vi "Ctr_FindRef[].vi"(5 "加入前缀(空)":string, 7 "ClassName(ALL)":string(combo), 8 "error in":errorcluster, 9 "结束字符串(_%)":string="_%", 10 "CtrlName[]":string[](array[string]), 11 "vi*(Current VI)":refnum<vi>) -> (0 "error out":errorcluster, 1 "CtrlLables[]":string[](array[string]), 2 "ctrls":refnum<vi>[](array[refnum]), 3 "vi* out":refnum<vi>)   [LabVIEW 2016]
uses:
  <vilib>/regexp/Match Regular Expression.xnode
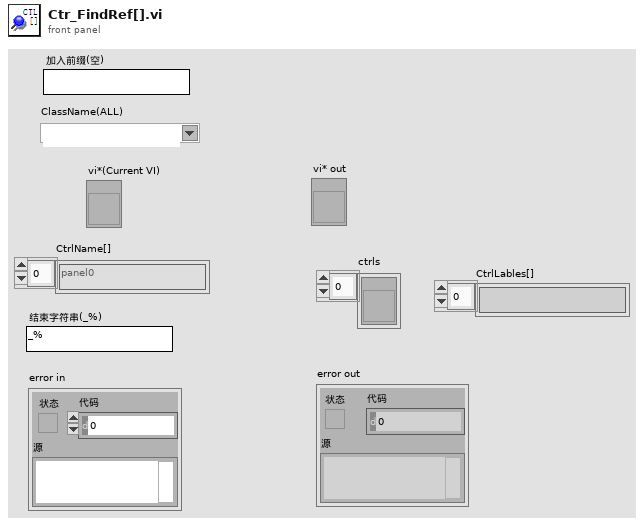
[diagram p1: front panel]
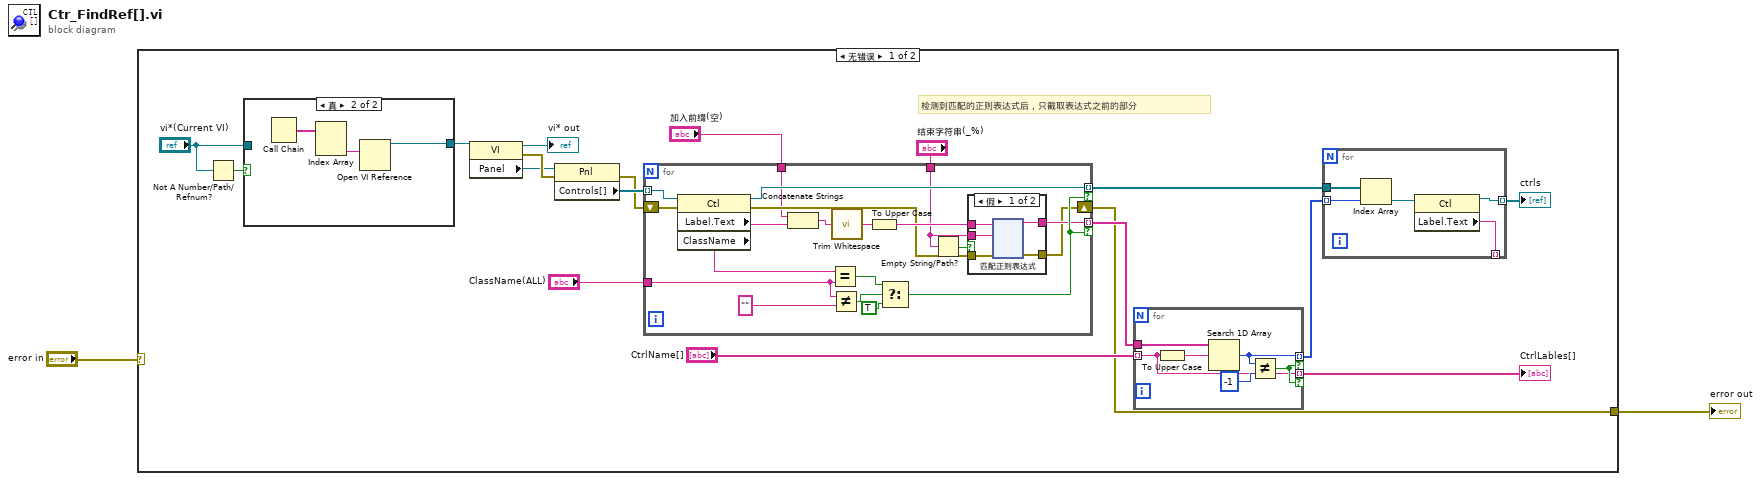
[diagram p0: block diagram]
diagram:
  n1 = case shown="无错误" "error in" {
    selector: "error in" -> [_ w177]
    tunnel: [w8 w177] -> w1
    frame No Error {
      # "检测到匹配的正则表达式后，只截取表达式之前的部分"
      n2 = Not A Number/Path/Refnum?(number/path/refnum="vi*(Current VI)") -> (NaN/Path/Refnum?=w15:bool)
      n3 = case shown="真" w15 {
        tunnel: [w32 w35] -> w16
        tunnel: "vi*(Current VI)" -> [w32 _]
        frame False {
        }
        frame True {
          n4 = Call Chain() -> (call chain=w34:string[])
          n5 = Index Array(array=w34) -> (element #2=w33:string)  [unwired: 2 in, 1 out]
          n6 = Open VI Reference(vi path=w33) -> (vi reference=w35:refnum<vi>)  [unwired: 5 in, 1 out]
        }
      }
      n7 = property class="VI"(reference=w16) -> (reference out=→"vi* out":refnum<vi>, error out=w19:errorcluster, "Panel"=w7:refnum<vi>)  [unwired: 1 in]
      n8 = property class="Pnl"(reference=w7, error in=w19) -> (error out=w18:errorcluster, "Controls[]"=w20:refnum<vi>[])  [unwired: 1 out]
      n9 = for {
        tunnel: w20 -> [w55] mode=indexing
        tunnel: [w54] -> w11 mode=indexing if=w46
        shift-right: [w41] -> w8
        shift-left: w18 -> [w53]
        tunnel: [w43] -> w13 mode=indexing if=w46
        tunnel: "ClassName(ALL)" -> [w50]
        tunnel: "结束字符串(_%)" -> [w40]
        tunnel: "加入前缀(空)" -> [w36]
        n10 = property class="Ctl"(reference=w55, error in=w53) -> (reference out=w54:refnum<vi>, error out=w42:errorcluster, "Label.Text"=w38:string, "ClassName"=w51:string)
        n11 = Concatenate Strings(w36, w38) -> (w37:string)
        n12 = Equal?(x=w51, y=w50) -> (x = y?=w47:bool)
        n13 = Not Equal?(x=w50, y="") -> (x != y?=w48:bool)
        n14 = call <vilib>:"Trim Whitespace.vi"("string"=w37) -> ("trimmed string"=w52:string)  [unwired: 1 in]
        n15 = To Upper Case(1:w52) -> (0:w44:string)
        n16 = Select(t=w47, s=w48, f=TRUE) -> (s? t:f=w46:bool)
        n17 = Empty String/Path?(string/path=w40) -> (empty?=w39:bool)
        n18 = case shown="假" w39 {
          tunnel: w44 -> [w60 w176]
          tunnel: [w59 w176] -> w43
          tunnel: w42 -> [w58 w175]
          tunnel: [w57 w175] -> w41
          tunnel: w40 -> [w56 _]
          frame False {
            n19 = xnode "匹配正则表达式"("输入字符串"=w60, "正则表达式"=w56, "错误输入"=w58) -> ("匹配之前"=w59:string, "错误输出"=w57:errorcluster)  [unwired: 3 in, 3 out]
          }
          frame True {
          }
        }
      }
      n20 = for {
        tunnel: w13 -> [w31]
        tunnel: "CtrlName[]" -> [w26] mode=indexing
        tunnel: [w30] -> w10 mode=indexing if=w28
        tunnel: [w26] -> w3 mode=indexing if=w28
        n21 = To Upper Case(1:w26) -> (0:w27:string)
        n22 = Search 1D Array(1D array=w31, element=w27) -> (index of element=w30:i32)  [unwired: 1 in]
        n23 = Not Equal?(x=w30, y=-1) -> (x != y?=w28:bool)
      }
      "CtrlLables[]" <- w3
      n24 = for {
        tunnel: w11 -> [w25]
        tunnel: w10 -> [w24] mode=indexing
        tunnel: [w22] -> w9 mode=indexing
        tunnel: [w21] -> _ mode=indexing
        n25 = Index Array(array=w25, index=w24) -> (element=w23:refnum<vi>)
        n26 = property class="Ctl"(reference=w23) -> (reference out=w22:refnum<vi>, "Label.Text"=w21:string)  [unwired: 1 in, 1 out]
      }
      "ctrls" <- w9
    }
    frame Error {
    }
  }
  "error out" <- w1
